vi "Load Device Info.vi"(8 "Error In":errorcluster, 11 "LINX Resource":T1) -> (0 "Error Out":errorcluster, 3 "LINX Resource":T1)   [LabVIEW 2019, in "LMH-LINX.lvlib" / "Local IO.lvlib"]
uses:
  <vilib>/MakerHub/LINX/Private/Local IO/Local IO.lvlib
  <vilib>/MakerHub/LINX/Private/Type Defs/LINX Ref.ctl
  <vilib>/MakerHub/LINX/Private/Type Defs/Platform.ctl
  <vilib>/MakerHub/LINX/Private/Type Defs/Interface.ctl
  <vilib>/MakerHub/LINX/Private/Device/Type Defs/LINX Device Config.ctl
  <vilib>/MakerHub/LINX/Private/Device/Type Defs/TCP Config.ctl
  <vilib>/MakerHub/LINX/Private/Device/Type Defs/Channels.ctl
  <vilib>/MakerHub/LINX/Private/Utilties/Generate Error.vi
  <vilib>/MakerHub/LINX/LMH-LINX.lvlib
  <vilib>/MakerHub/LINX/Private/Device/Device.lvlib
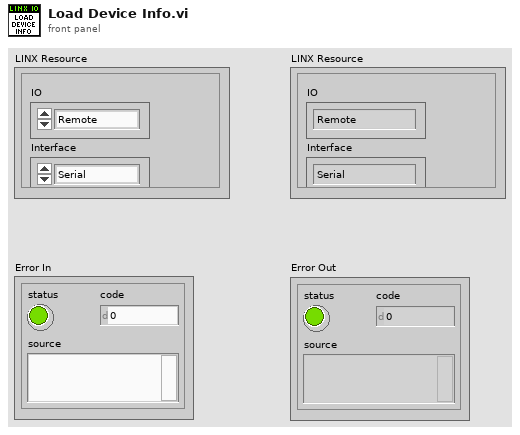
[diagram p1: front panel]
types:
  T1 = typedef "LMH-LINX.lvlib/LINX Ref.ctl" = cluster{"IO":T2, "Interface":T3, "LINX Device Config":T4}
  T2 = typedef "LMH-LINX.lvlib/Platform.ctl" = enum16{"Remote", "Local"}
  T3 = typedef "LMH-LINX.lvlib/Interface.ctl" = enum16{"Serial", "TCP"}
  T4 = typedef "LMH-LINX.lvlib/Device.lvlib/LINX Device Config.ctl" = cluster{"Interface":T3, "COM Port":refnum<visa-resource-name>, "TCP Configuration":T5, "Device Family":u8, "Device ID":u8, "Device Name":string, "TCP Ref":refnum<k5>, "Channels":T6}
  T5 = typedef "LMH-LINX.lvlib/Device.lvlib/TCP Config.ctl" = cluster{"IP Address":string, "Port":u16}
  T6 = typedef "LMH-LINX.lvlib/Channels.ctl" = cluster{"DI":u8[], "DO":u8[], "AI":u8[], "AO":u8[], "PWM":u8[], "QE":u8[], "UART":u8[], "I2C 2":u8[], "SPI":u8[], "CAN":u8[], "Servo":u8[], "AI Ref (V)":dbl, "AI Resolution (Bits)":u8, "AO Ref (V)":dbl, "AO Resolution (Bits)":u8}
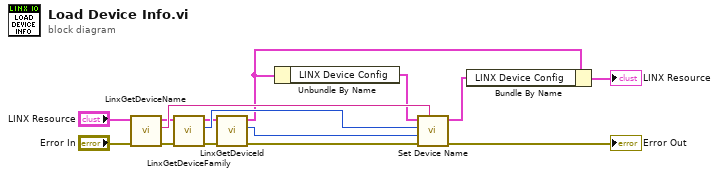
[diagram p0: block diagram]
diagram:
  n1 = call <vilib>:"LinxGetDeviceName.vi"("Error In"="Error In", "LINX Resource"="LINX Resource") -> ("Error Out"=w9:errorcluster, "Device Name"=w13:string, "LINX Resource"=w8:T1)  [unwired: 7 in]
  n2 = call <vilib>:"LinxGetDeviceFamily.vi"("Error In"=w9, "LINX Resource"=w8) -> ("Error Out"=w11:errorcluster, "DeviceFamily"=w14:u8, "LINX Resource"=w10:T1)  [unwired: 7 in]
  n3 = call <vilib>:"LinxGetDeviceId.vi"("Error In"=w11, "LINX Resource"=w10) -> ("Error Out"=w12:errorcluster, "DeviceID"=w15:u8, "LINX Resource"=w1:T1)  [unwired: 7 in]
  n4 = Unbundle By Name(w1) -> ("LINX Device Config"=w5:T4)
  n5 = call <vilib>:"Set Device Name.vi"("Device Name"=w13, "Error In"=w12, "Device ID"=w15, "Device Family"=w14, "LINX Device Config"=w5) -> ("Error Out"=→"Error Out":errorcluster, "LINX Device Config"=w6:T4)  [unwired: 5 in]
  n6 = Bundle By Name(cluster=w1, "LINX Device Config"=w6) -> (→"LINX Resource":T1)
